vi "FpgaLink_Play_XSVF.vi"(8 "error in (no error)":errorcluster, 10 "xsvf file":path, 11 "handle":i64) -> (0 "error out":errorcluster, 3 "handle out":i64)   [LabVIEW 2011]
doc: "Play an SVF, XSVF or CSVF file into the JTAG chain.\n\nDespite the name of the function, it does actually support regular Serial Vector Format files and Compressed Serial Vector Format files in addition to Xilinx Serial Vector Format files. All are simply played into the JTAG chain, so it's your responsibility to ensure that the file is created for the appropriate chain configuration. Typically, this is used for programming devices, but it doesn't have to be - the file can be arbitrary JTAG operations. Before calling flPlayXSVF(), you should verify that the FPGALink device actually supports NeroJTAG using flIsNeroCapable()."
uses:
  <vilib>/Utility/importsl/GetValueByPointer/datatype.ctl
  <vilib>/Utility/importsl/GetValueByPointer/GetValueByPointer.xnode
  resource/lvimptsl.dll
  libfpgalink.dll
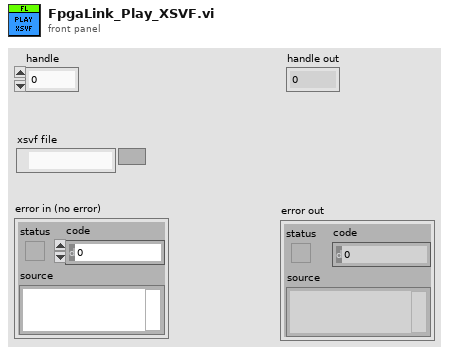
[diagram p1: front panel]
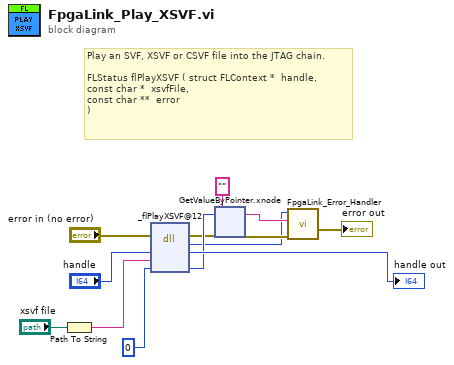
[diagram p0: block diagram]
diagram:
  # "Play an SVF, XSVF or CSVF file into the JTAG chain.\n\nFLStatus flPlayXSVF\t(\tstruct FLContext * \thandle,\nconst char * \txsvfFile,\nconst char ** \terror \n)"
  n1 = Path To String(path="xsvf file") -> (string=w7:string)
  n2 = dll-call lib="libfpgalink.*" fn="_flPlayXSVF@12"(error in="error in (no error)", "handle"="handle", "xsvfFile"=w7, "error"=i64 0) -> (error out=w8:errorcluster, "FLStatus"=w2:u32, "handle"=→"handle out":i64, "error"=w9:i64)  [unwired: 3 in, 1 out]
  n3 = xnode "GetValueByPointer.xnode"("Pointer"=w9, "InputType"="", "ErrorIn"=w8) -> ("Output"=w3:string, "ErrorOut"=w4:errorcluster)  [unwired: 1 in]
  n4 = call <vilib>:"FpgaLink_Error_Handler.vi"("error in (no error)"=w4, "error string"=w3, "error code"=w2) -> ("error out"=→"error out":errorcluster)  [unwired: 8 in]
